vi "projetoIM_labview2021-matebookx.vi"() -> ()   [LabVIEW 2021]
uses:
  <vilib>/express/express arith-compare/Formula/XNode/ExpressFormulaBlockNode.xnode
  <vilib>/express/express shared/transition.llb/Dynamic To Waveform Array.vi
  <vilib>/express/express arith-compare/Formula/Block/exnFormulaBlock how many pts in the wave.vi
  <vilib>/express/express shared/ex_Modify Signal Name.vi
  <vilib>/express/express shared/transition.llb/Waveform Array To Dynamic.vi
panel:
  out "Numeric":dbl
  out "Vout":dbl
  in  "stop":bool
  out "data":dynamicdata(graph)
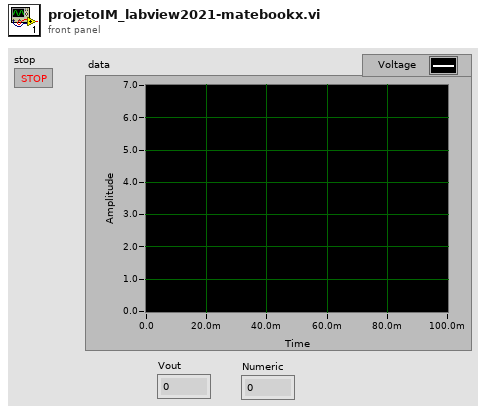
[diagram p1: front panel]
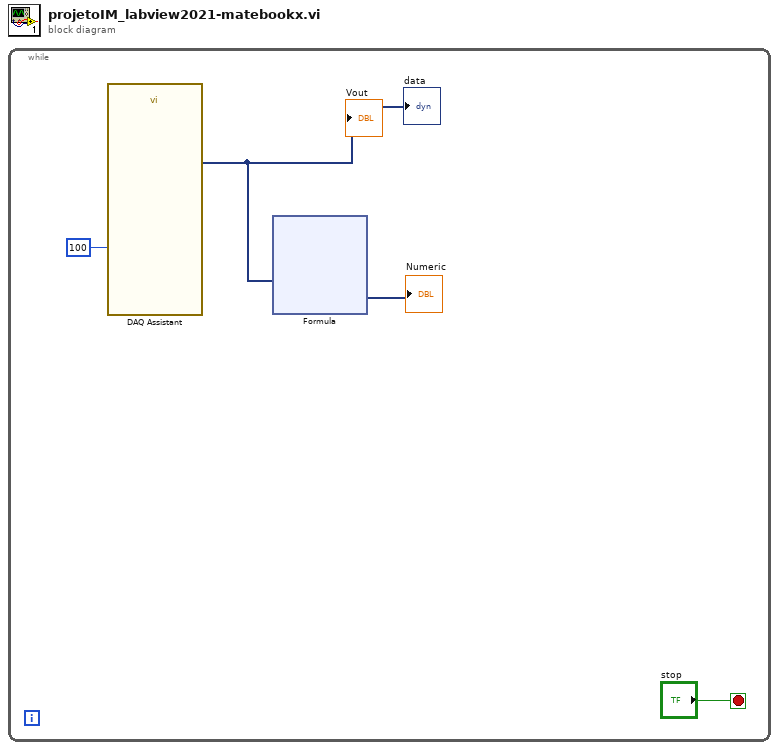
[diagram p0: block diagram]
diagram:
  n1 = while {
    stop <- "stop" stop-if-true
    n2 = call "DAQ Assistant"("number of samples"=100) -> ("data"=w2:dynamicdata)  [unwired: 16 in, 2 out]
    "data" <- w2
    "Vout" <- w2
    n3 = xnode "Formula"("X1"=w2) -> ("Result"=→"Numeric":dynamicdata)  [unwired: 1 in, 1 out]
  }
